vi "M30XYConnectSetVelocityStep.vi"() -> ()   [LabVIEW 2015]
uses:
  C:/Users/fmovagharnemati/OneDrive - THORLABS Inc/Desktop/github/M30XY/Thorlabs.MotionControl.Controls.dll
  github/M30XY/Thorlabs.MotionControl.Controls.dll
  C:/Users/fmovagharnemati/OneDrive - THORLABS Inc/Desktop/github/M30XY/ThorLabs.MotionControl.Benchtop.DCServoCLI.dll
  github/M30XY/ThorLabs.MotionControl.Benchtop.DCServoCLI.dll
panel:
  in  "stepSize":dbl
  in  "direction":i32(ring)=1 items=["Forward"=1, "Backward"=2]
  in  "acceleration":dbl
  in  "maxVelocity":dbl
  in  "Channel Number":i32=1
  in  "?":bool
  in  "Set Velocity Params":bool
  in  "Move Relative":bool
  in  "Home":bool
  in  "SerialNumber":string
  in  "BenchtopDCServoControl":refnum<k24>(container)
  # "Thorlabs Hardware: M30XY - 30 mm Motorized XY Translation Stage\nhttps://www.thorlabs.com/thorproduct.cfm?partnumber=M30XY\n\nDescription: This VI will enable you to communicate with M30XY series to control  Brushless Stages & Actuators. \n\nInstructions: \n1) Connect your M30XY  device to your PC & power the device, ensuring your stage/actutator is connected. For full device setup, the device product manual can be found on our website.\n2) Enter the device serial number.\n3) Click 'Run' in the LabVIEW Toolbar which will attempt a connection, and enable the device.\n4) Ensure the device move path is clear for homing, and press Home.\n5) Await for device to be be available, and to have finished homing (Home indicator in control panel should be green).\n6) Input direction and step size for relative move.\n7) To end the Program click 'STOP'."
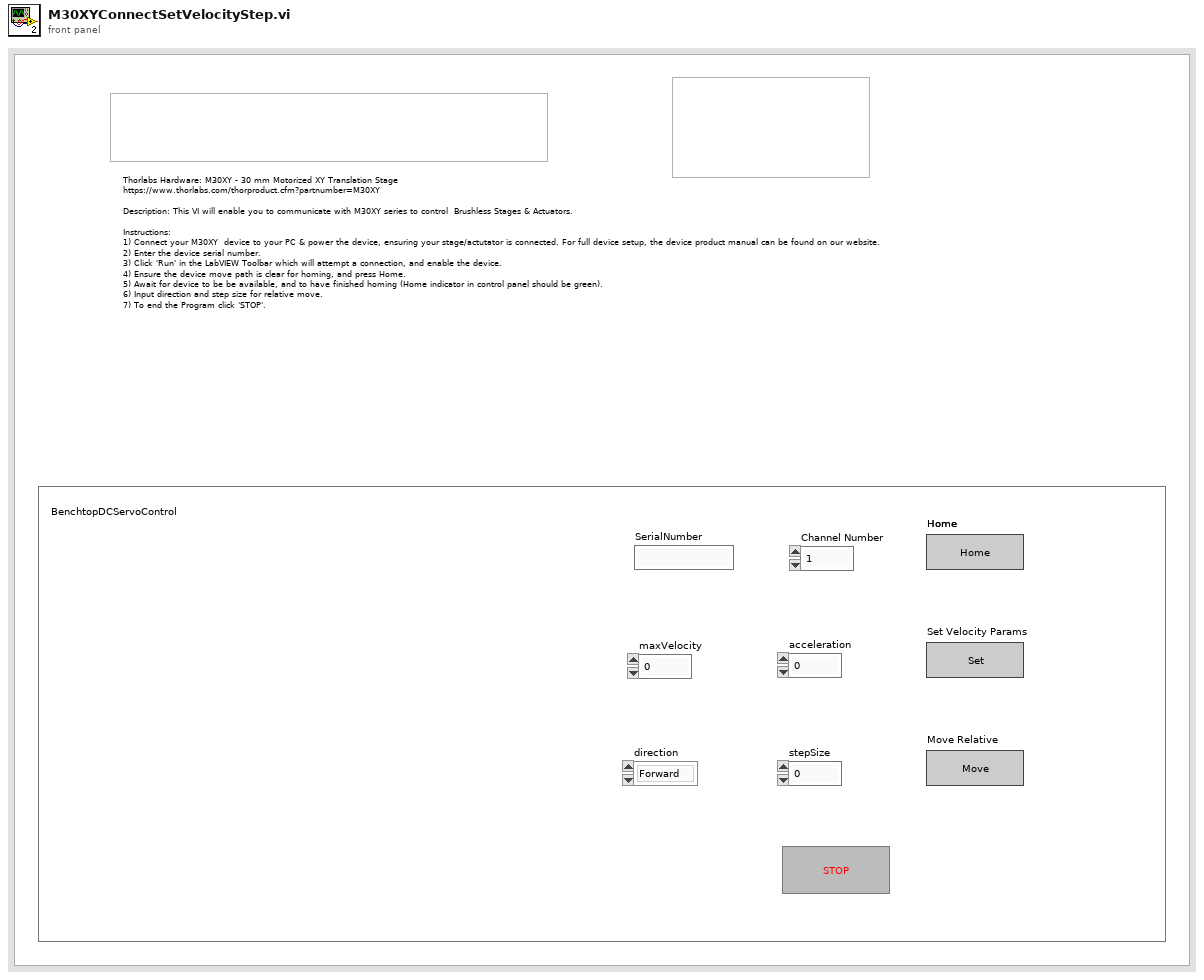
[diagram p1: front panel]
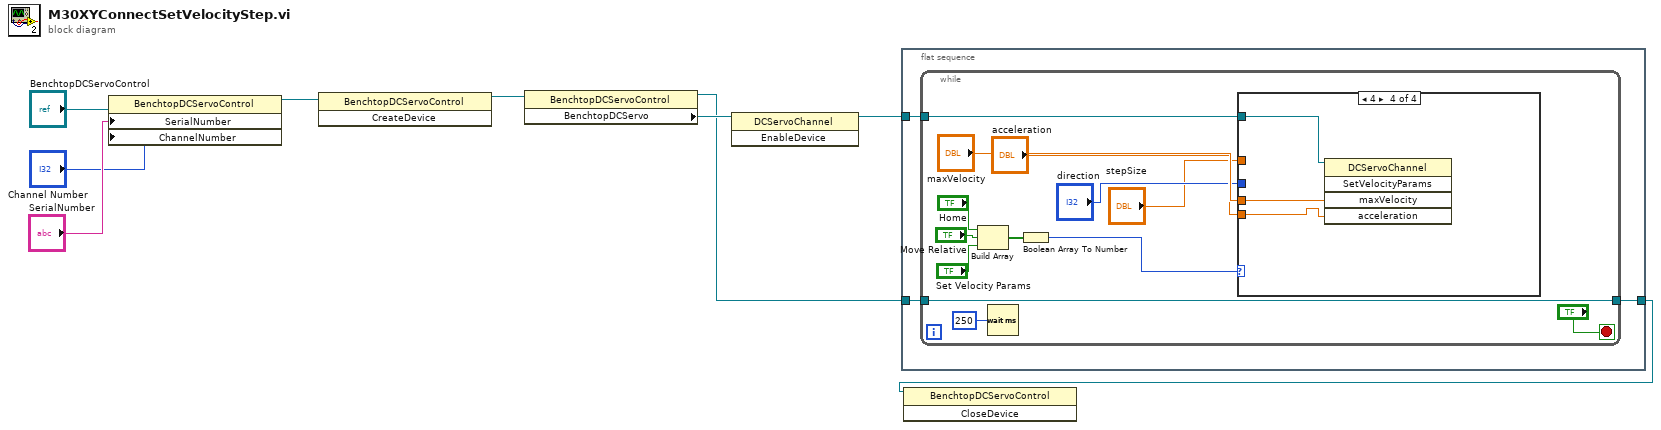
[diagram p0: block diagram]
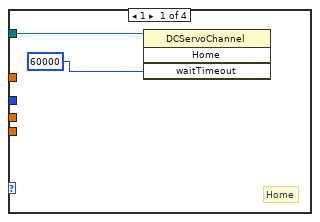
[diagram p2: hidden frame]
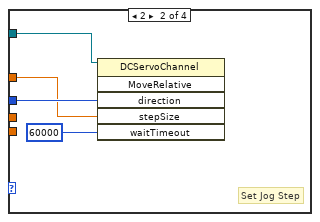
[diagram p3: hidden frame]
diagram:
  n1 = property class="BenchtopDCServoControl"(reference="BenchtopDCServoControl", "SerialNumber"="SerialNumber", "ChannelNumber"="Channel Number") -> (reference out=w7:refnum<k24>)  [unwired: 1 in, 1 out]
  n2 = invoke class="BenchtopDCServoControl" method="CreateDevice"(reference=w7) -> (reference out=w6:refnum<k24>)  [unwired: 2 in, 2 out]
  n3 = property class="BenchtopDCServoControl"(reference=w6) -> (reference out=w3:refnum<k24>, "BenchtopDCServo"=w4:refnum<k24>)  [unwired: 1 in, 1 out]
  n4 = invoke class="DCServoChannel" method="EnableDevice"(reference=w4) -> (reference out=w2:refnum<k24>)  [unwired: 2 in, 2 out]
  n5 = flat-sequence {
    tunnel: w3 -> [w12]
    tunnel: [w11] -> w1
    tunnel: w2 -> [w10]
    frame #0 {
      n6 = while {
        tunnel: [w18] -> w11
        tunnel: w10 -> [w21]
        tunnel: w12 -> [w18]
        stop <- "?" stop-if-true
        n7 = Build Array("Home", "Move Relative", "Set Velocity Params") -> (w20:bool[])
        n8 = Wait (ms)(milliseconds to wait=u32 250) -> ()  [unwired: 1 out]
        n9 = Boolean Array To Number(Boolean array=w20) -> (number=w19:u32)
        n10 = case shown="4" w19 {
          tunnel: w21 -> [w26 w31 _ w32]
          tunnel: "maxVelocity" -> [_ _ _ w34]
          tunnel: "acceleration" -> [_ _ _ w33]
          tunnel: "direction" -> [_ w30 _ _]
          tunnel: "stepSize" -> [_ w29 _ _]
          frame 1 {
            # "Home"
            n11 = invoke class="DCServoChannel" method="Home"(reference=w26, "waitTimeout"=60000) -> ()  [unwired: 2 in, 4 out]
          }
          frame 2 {
            # "Set Jog Step"
            n12 = invoke class="DCServoChannel" method="MoveRelative"(reference=w31, "direction"=w30, "stepSize"=w29, "waitTimeout"=60000) -> ()  [unwired: 2 in, 6 out]
          }
          frame Default {
          }
          frame 4 {
            n13 = invoke class="DCServoChannel" method="SetVelocityParams"(reference=w32, "maxVelocity"=w34, "acceleration"=w33) -> ()  [unwired: 2 in, 5 out]
          }
        }
      }
    }
  }
  n14 = invoke class="BenchtopDCServoControl" method="CloseDevice"(reference=w1) -> ()  [unwired: 2 in, 3 out]
